vi "Parse All Structure Data.vi"(8 "Error In":errorcluster, 9 "Data":string, 10 "Structure IDs":string[](array[string]), 11 "Nest Config":T1) -> (0 "Error Out":errorcluster, 1 "Data":string, 2 "Structures":T4[](array[typedef]), 3 "Nest Config":T1)   [LabVIEW 2013, in "LMH-Nest.lvlib"]
uses:
  LMH-Nest.lvlib
  Type Defs/Structure.ctl
  Type Defs/Nest Config.ctl
  <vilib>/httpClient/ClientHandle.ctl
  Type Defs/Session Data.ctl
  <vilib>/httpClient/LabVIEWHTTPClient.lvlib
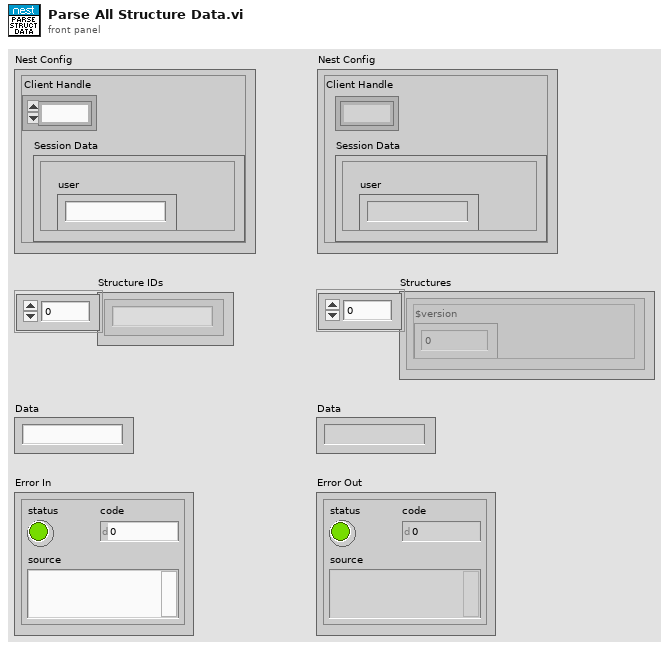
[diagram p1: front panel]
types:
  T1 = typedef "LMH-Nest.lvlib/Nest Config.ctl" = cluster{"Client Handle":T2, "Session Data":T3}
  T2 = typedef "LabVIEWHTTPClient.lvlib/ClientHandle.ctl" = refnum<k1>
  T3 = typedef "LMH-Nest.lvlib/Session Data.ctl" = cluster{"is_superuser":bool, "is_staff":bool, "urls":cluster{"transport_url":string, "rubyapi_url":string, "weather_url":string, "log_upload_url":string, "support_url":string}, "limits":cluster{"thermostats_per_structure":u32, "structures":u32, "thermostats":u32, "smoke_detectors":u32, "smoke_detectors_per_structure":u32}, "access_token":string, "userid":string, "expires_in":string, "email":string, "user":string, "language":string}
  T4 = typedef "LMH-Nest.lvlib/Structure.ctl" = cluster{"$version":i32, "$timestamp":dbl, "dr_reminder_enabled":bool, "renovation_date":string, "country_code":string, "hvac_safety_shutoff_enabled":bool, "away":bool, "house_type":string, "topaz_enhanced_auto_away_enabled":bool, "name":string, "postal_code":string, "creation_time":dbl, "num_thermostats":string, "away_setter":dbl, "structure_area":dbl, "user":string, "devices":string[], "swarm":string[], "fabric_ids":string[]}
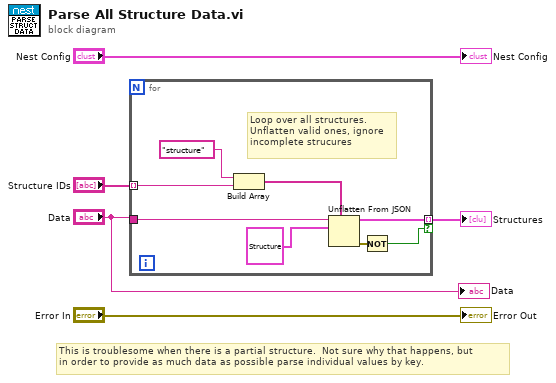
[diagram p0: block diagram]
diagram:
  # "This is troublesome when there is a partial structure.  Not sure why that happens, but \nin order to provide as much data as possible parse individual values by key."
  n1 = for {
    tunnel: [w10] -> w5 mode=indexing if=w8
    tunnel: "Data" -> [w7]
    tunnel: "Structure IDs" -> [w6] mode=indexing
    # "Loop over all structures.\nUnflatten valid ones, ignore\nincomplete strucures"
    n2 = Build Array("structure", w6) -> (w11:string[])
    n3 = Unflatten From JSON(path=w11, JSON string=w7, type and defaults=T4 {"$version"=0, "$timestamp"=0.0, "dr_reminder_enabled"=FALSE, "renovation_date"="", "country_code"="", "hvac_safety_shutoff_enabled"=FALSE, "away"=FALSE, "house_type"="", "topaz_enhanced_auto_away_enabled"=FALSE, "name"="", "postal_code"="", "creation_time"=0.0, "num_thermostats"="", "away_setter"=0.0, "structure_area"=0.0, "user"="", "devices"=[], "swarm"=[], "fabric_ids"=[]} ("Structure")) -> (value=w10:T4, error out=w9:errorcluster)  [unwired: 4 in]
    n4 = Not(x=w9) -> (.not. x?=w8:bool)
  }
  "Structures" <- w5
  "Error Out" <- "Error In"
  "Nest Config" <- "Nest Config"
  "Data" <- "Data"
